vi "uActor_Core.vi"(8 "error in (no error)":errorcluster, 11 "uBroker in":refnum<class "uBroker.lvclass">) -> (0 "error out":errorcluster, 3 "uBroker out":refnum<class "uBroker.lvclass">)   [LabVIEW 2021, in "uFramework.lvlib" / "uBroker.lvclass"]
uses:
  uBroker.lvclass
  U:/Projects/LABME/Src/uFramework/uActor/uActor.lvclass
  uMsg/uMsg.lvclass
  uMsg/uMsg.lvclass/uMsg.ctl
  uBroker.lvclass/uBroker.ctl
  uActor/uActor.lvclass/uActor.ctl
  uClient/uClient.lvclass/uClient.ctl
  uClient_Subscriber/uClient_Subscriber.lvclass/uClient_Subscriber.ctl
  uPolicy/uPolicy.lvclass/uPolicy.ctl
  uSubscription/uSubscription.lvclass/uSubscription.ctl
  uNotifyMode/uNotifyMode.lvclass/uNotifyMode.ctl
  uTransport_uActor/uTransport_uActor.lvclass/uTransport_uActor.ctl
  uTransport_Event/uTransport_Event.lvclass/uTransport_Event.ctl
  uTransport_Queue/uTransport_Queue.lvclass/uTransport_Queue.ctl
  uSubscription/uSubscription Create.vi
  uSubscription/uSubscription Update.vi
  uMsg/uMsg Get CMD.vi
  uClient_Publisher/uPublisher IsAlive.vi
  uSubscription/uSubscription IsAlive.vi
  uTransport_uActor/uTransport_uActor_SendMsg.vi
  uMsg/uMsg Get Payload.vi
  uClient/uClient_GetTransport.vi
  uClient_Subscriber/uSubscriber Get uPolicy.vi
  uPolicy/Read uNotifyMode.vi
  uPolicy/Read uStringManipulation.vi
  uNotifyMode/uNotify Update.vi
  uMsg/uMsg Rename CMD.vi
  uTransport/uTransport_SendMsg.vi
  uTransport_Event/uTransport_Event_SendMsg.vi
  uTransport_Queue/uTransport_Queue_SendMsg.vi
  uMsg/uMsg Update Timestamp.vi
  uClient_Subscriber/uClient_Subscriber.lvclass
  U:/Projects/LABME/Src/uFramework/uClient/uClient.lvclass
  uClient_Publisher/uClient_Publisher.lvclass
  Bin/uData.lvlibp/Get Tag.vi
  Bin/uData.lvlibp/Set Tag.vi
  uActor/uActor.lvclass
  Bin/uData.lvlibp/uData.lvclass
  uTransport/uTransport.lvclass
  uSubscription/uSubscription.lvclass
  uPolicy/uPolicy.lvclass
  uNotifyMode/uNotifyMode.lvclass
  uStringManipulation/uStringManipulation.lvclass
  uTransport_uActor/uTransport_uActor.lvclass
  uTransport_Event/uTransport_Event.lvclass
  uTransport_Queue/uTransport_Queue.lvclass
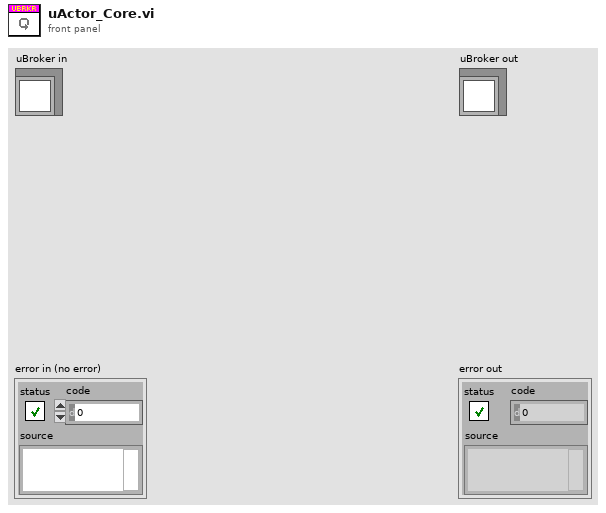
[diagram p1: front panel]
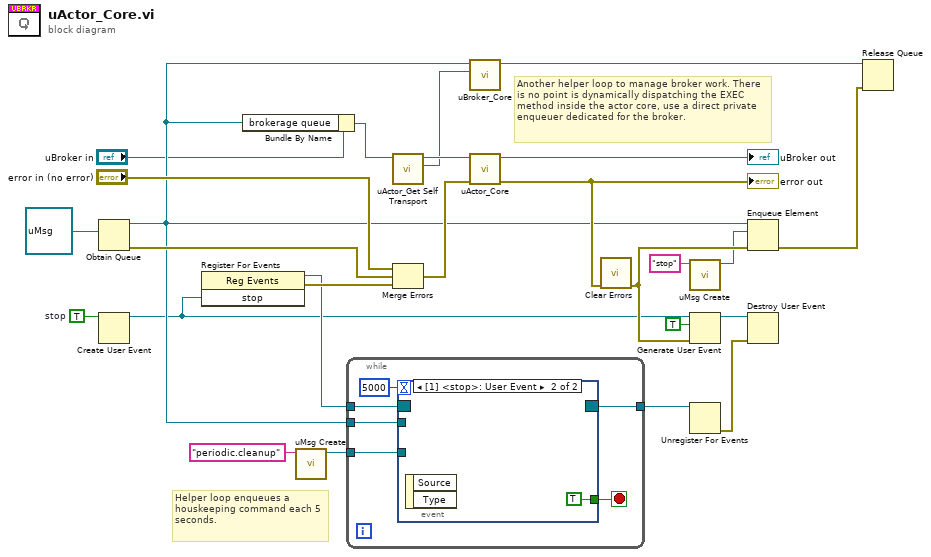
[diagram p0: block diagram]
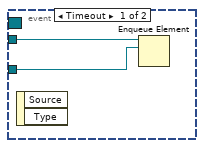
[diagram p2: hidden frame]
diagram:
  w21 = TRUE  # stop
  # "Another helper loop to manage broker work. There is no point is dynamically dispatching the EXEC method inside the actor core, use a direct private enqueuer dedicated for the broker."
  # "Helper loop enqueues a houskeeping command each 5 seconds."
  n1 = Obtain Queue(element data type=refnum<class "uMsg.lvclass"> refnum ("uTransport.lvlib:uMsg.lvclass")) -> (queue out=w10:refnum<queue>, error out=w26:errorcluster)  [unwired: 4 in, 1 out]
  n2 = Create User Event(user event datatype=w21) -> (user event=w8:refnum<user-event>)  [unwired: 1 in, 1 out]
  n3 = register-events(w8) -> (reference out=w20:refnum<event-registration>, error out=w23:errorcluster)  [unwired: 2 in]
  n4 = Bundle By Name(cluster="uBroker in", "brokerage queue"=w10) -> (w7:refnum<class "uBroker.lvclass">)
  n5 = call "uMsg Create.vi"("CMD"="periodic.cleanup") -> ("uMsg out"=w12:refnum<class "uMsg.lvclass">)  [unwired: 9 in, 1 out]
  n6 = while {
    tunnel: w20 -> [w32]
    tunnel: [w31] -> w19
    tunnel: w10 -> [w28]
    tunnel: w12 -> [w27]
    stop <- w29 stop-if-true
    n7 = event shown="[1] <stop>: User Event" {
      selector: w32 -> [_ _]
      dyn-events: [_ _] -> w31
      timeout: 5000 -> [_ _]
      tunnel: [_ TRUE] -> w29
      tunnel: w28 -> [w34 _]
      tunnel: w27 -> [w33 _]
      event Timeout {
        n8 = event-data() -> ()  [unwired: 1 in, 2 out]
        n9 = Enqueue Element(queue=w34, element=w33) -> ()  [unwired: 2 in, 3 out]
      }
      event User Event {
        n10 = event-data() -> ()  [unwired: 1 in, 2 out]
      }
    }
  }
  n11 = call "uActor_Get Self Transport.vi"("uActor in"=w7) -> ("Actor Transport"=w1:refnum<class "uTransport_uActor.lvclass">, "uActor out"=w2:refnum<class "uBroker.lvclass">)  [unwired: 9 in]
  n12 = Merge Errors("error in (no error)", w26, w23) -> (w15:errorcluster)
  n13 = call "uBroker_Core.vi"("ActorCore Transport"=w1, "brokerage queue in"=w10) -> ("brokerage queue out"=w4:refnum<queue>)  [unwired: 9 in]
  n14 = call-parent "uActor_Core.vi"("error in (no error)"=w15, "uActor in"=w2) -> ("error out"=w18:errorcluster, "uActor out"=→"uBroker out":refnum<class "uBroker.lvclass">)  [unwired: 8 in]
  "error out" <- w18
  n15 = call <vilib>:"Clear Errors.vi"("error in (no error)"=w18) -> ("error out"=w24:errorcluster)  [unwired: 5 in, 1 out]
  n16 = call "uMsg Create.vi"("CMD"="stop") -> ("uMsg out"=w6:refnum<class "uMsg.lvclass">)  [unwired: 9 in, 1 out]
  n17 = Generate User Event(user event=w8, event data cluster=TRUE ("event data"), error in=w24) -> (user event out=w17:refnum<user-event>)  [unwired: 1 in, 1 out]
  n18 = Unregister For Events(event registration refnum=w19) -> (error out=w16:errorcluster)  [unwired: 1 in]
  n19 = Enqueue Element(queue=w10, element=w6, error in (no error)=w24) -> (error out=w3:errorcluster)  [unwired: 1 in, 2 out]
  n20 = Destroy User Event(user event=w17, error in=w16) -> ()  [unwired: 1 out]
  n21 = Release Queue(queue=w4, error in (no error)=w3) -> ()  [unwired: 1 in, 3 out]
